vi "Autosize Reshape 2D String Array.vi"(10 "Array in":string[][](array[string])) -> (2 "Array out":string[][](array[string]))   [LabVIEW 2015]
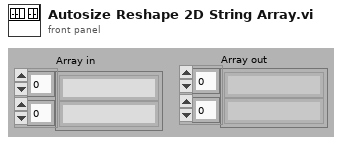
[diagram p1: front panel]
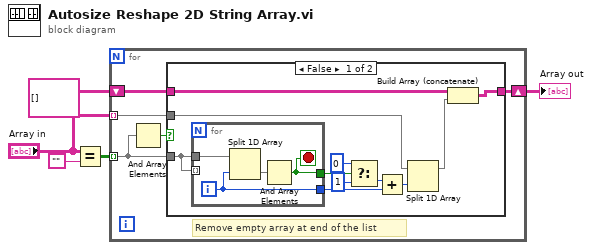
[diagram p0: block diagram]
diagram:
  n1 = Equal?(x="Array in", y="") -> (x = y?=w3:bool[][])
  n2 = for {
    tunnel: w3 -> [w7] mode=indexing
    tunnel: "Array in" -> [w10] mode=indexing
    shift-right: [w9] -> w1
    shift-left: string[][] [] -> [w8]
    # "Remove empty array at end of the list"
    n3 = And Array Elements(Boolean array=w7) -> (logical AND=w6:bool)
    n4 = case shown="False" w6 {
      tunnel: w10 -> [w21 _]
      tunnel: w7 -> [w20 _]
      tunnel: [w19 w26] -> w9
      tunnel: w8 -> [w18 w26]
      frame False {
        n5 = for {
          tunnel: w20 -> [w25]
          tunnel: w20 -> [_] mode=indexing
          tunnel: [w24] -> w12
          tunnel: [w22] -> w16
          i -> [w24]
          stop <- w22 stop-if-true
          n6 = Split 1D Array(array=w25, index=w24) -> (second subarray=w23:bool[])  [unwired: 1 out]
          n7 = And Array Elements(Boolean array=w23) -> (logical AND=w22:bool)
        }
        n8 = Select(t=0, s=w16, f=1) -> (s? t:f=w13:i32)
        n9 = Add(x=w13, y=w12) -> (x+y=w11:i32)
        n10 = Split 1D Array(array=w21, index=w11) -> (first subarray=w17:string[])  [unwired: 1 out]
        n11 = Build Array (concatenate)(w18, w17) -> (w19:string[][])
      }
      frame True {
      }
    }
  }
  "Array out" <- w1
